vi "5.4.vi"() -> ()   [LabVIEW 2017]
panel:
  out "任务四":string
  # "【加入了延时】"
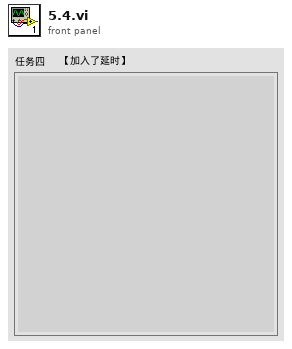
[diagram p1: front panel]
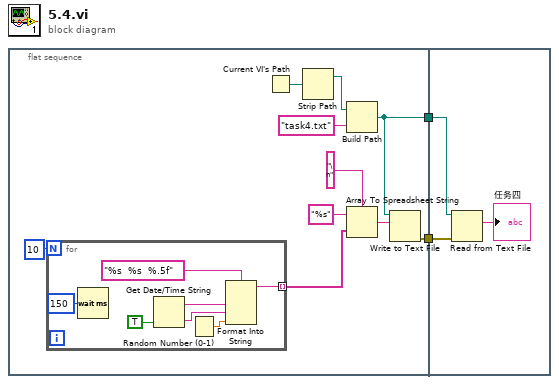
[diagram p0: block diagram]
diagram:
  n1 = flat-sequence {
    tunnel: [w4] -> w2
    tunnel: [w3] -> w1
    tunnel: w2 -> [w21]
    tunnel: w1 -> [w20]
    frame #0 {
      n2 = for {
        N: 10 -> [_]
        tunnel: [w17] -> w9 mode=indexing
        n3 = Wait (ms)(milliseconds to wait=u32 150 ("等待时间（毫秒）")) -> ()  [unwired: 1 out]
        n4 = Get Date/Time String(want seconds? (F)=TRUE) -> (date string=w18:string, time string=w14:string)  [unwired: 2 in]
        n5 = Random Number (0-1)() -> (number: 0 to 1=w15:dbl)
        n6 = Format Into String(format string="%s  %s  %.5f" ("格式字符串"), w18, w14, w15) -> (resulting string=w17:string)  [unwired: 2 in, 1 out]
      }
      n7 = Current VI's Path() -> (path=w11:path)
      n8 = Strip Path(path=w11) -> (stripped path=w12:path)  [unwired: 1 out]
      n9 = Build Path(base path=w12, name or relative path="task4.txt") -> (appended path=w4:path)
      n10 = Array To Spreadsheet String(delimiter (Tab)="\n" ("分隔符(Tab)"), array=w9, 3:"%s" ("格式字符串")) -> (spreadsheet string=w10:string)
      n11 = Write to Text File(file (use dialog)=w4, text=w10) -> (error out=w3:errorcluster)  [unwired: 2 in, 2 out]
    }
    frame #1 {
      n12 = Read from Text File(file (use dialog)=w21, error in=w20) -> (text=→"任务四":string)  [unwired: 2 in, 3 out]
    }
  }
